vi "picoquant_set_channel.vi"(8 "error in (no error)":errorcluster, 9 "channel_num":i32, 10 "ch_settings":T1 {"ch_offs" min=-99999 max=99999 step=1; "ch_ZeroX" min=0 max=20 step=1; "ch_level" min=0 max=800 step=10}, 11 "picoharp in":refnum<class "picoharp.lvclass">) -> (0 "error out":errorcluster, 3 "picoharp out":refnum<class "picoharp.lvclass">)   [LabVIEW 2015, in "picoharp.lvclass"]
uses:
  picoharp.lvclass
  Hydraharp/hydraharp_panel/hpanel_channel_settings.ctl
  picoharp.lvclass/picoharp.ctl
  phlib.dll
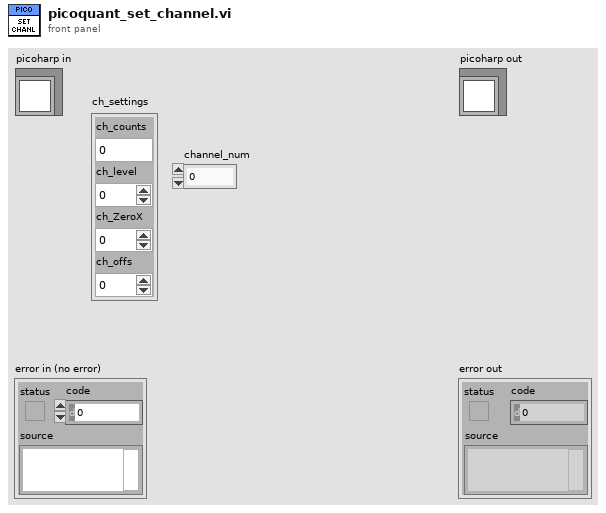
[diagram p1: front panel]
types:
  T1 = typedef "hpanel_channel_settings.ctl" = cluster{"ch_counts":i32, "ch_level":i32, "ch_ZeroX":i32, "ch_offs":i32}
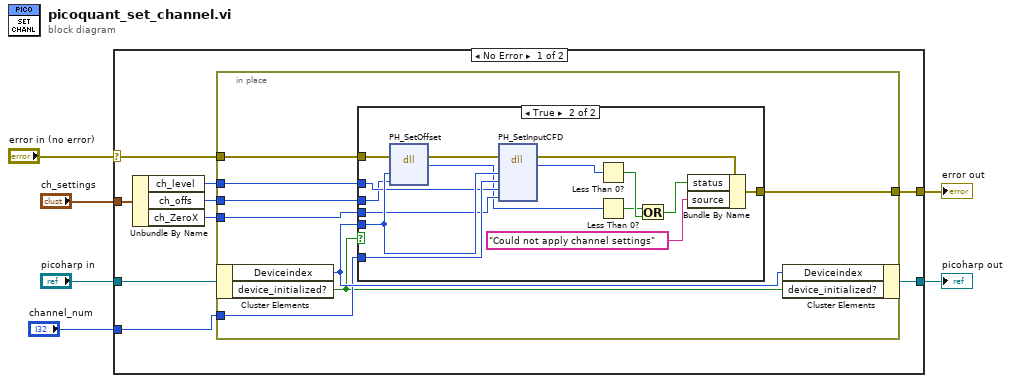
[diagram p0: block diagram]
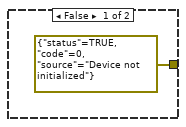
[diagram p2: hidden frame]
diagram:
  n1 = case shown="No Error" "error in (no error)" {
    selector: "error in (no error)" -> [w8 w41]
    tunnel: [w7 w41] -> w2
    tunnel: [w9 w40] -> w1
    tunnel: "picoharp in" -> [w15 w40]
    tunnel: "ch_settings" -> [w13 _]
    tunnel: "channel_num" -> [w14 _]
    frame No Error {
      n2 = Unbundle By Name(w13) -> ("ch_level"=w12:i32, "ch_offs"=w11:i32, "ch_ZeroX"=w10:i32)
      n3 = in-place {
        in-place-border: w14 -> [w22]
        in-place-border: w12 -> [w21]
        in-place-border: w11 -> [w20]
        in-place-border: w10 -> [w19]
        in-place-border: w8 -> [w17]
        in-place-border: [w18] -> w7
        n4 = in-place-cluster #1(w15) -> ("Deviceindex"=w23:i32, "device_initialized?"=w16:bool)
        n5 = case shown="True" w16 {
          tunnel: w23 -> [_ w39]
          tunnel: w22 -> [_ w38]
          tunnel: w21 -> [_ w37]
          tunnel: w20 -> [_ w25]
          tunnel: w19 -> [_ w36]
          tunnel: [errorcluster {"status"=TRUE, "code"=0, "source"="Device not initialized"} ("error IO") w26] -> w18
          tunnel: w17 -> [_ w31]
          frame False {
          }
          frame True {
            n6 = dll-call lib="phlib.dll" fn="PH_SetOffset" label="pH_Setoffset"(error in=w31, "devidx"=w39, "offset"=w25) -> (error out=w30:errorcluster, "return type"=w35:i32)  [unwired: 4 in, 1 out]
            n7 = dll-call lib="phlib.dll" fn="PH_SetInputCFD" label="pH_SetInputCFD"(error in=w30, "devidx"=w39, "channel"=w38, "level"=w37, "zerox"=w36) -> (error out=w29:errorcluster, "return type"=w34:i32)  [unwired: 6 in, 1 out]
            n8 = Less Than 0?(x=w34) -> (x < 0?=w33:bool)
            n9 = Less Than 0?(x=w35) -> (x < 0?=w32:bool)
            n10 = Or(x=w32, y=w33) -> (x .or. y?=w28:bool)
            n11 = Bundle By Name(cluster=w29, "status"=w28, "source"="Could not apply channel settings") -> (w26:errorcluster)
          }
        }
        n12 = in-place-cluster #1("Deviceindex"=w23, "device_initialized?"=w16) -> (w9:refnum<class "picoharp.lvclass">)
      }
    }
    frame Error {
    }
  }
  "error out" <- w2
  "picoharp out" <- w1
